vi "Get ixon camera info.vi"() -> ()   [LabVIEW 2011]
uses:
  <userlib>/atmcd32d.llb/HSSpeed_type typedef.ctl
  <userlib>/atmcd32d.llb/AndorCapabilities typedef.ctl
panel:
  out "Preamp gains":sgl[](array[numeric])
  out "# y pixels":i32
  out "# x pixels":i32
  out "highest EM gain":i32
  out "lowest EM gain":i32
  out "camera serial #":i32
  out "Flex version #":u32
  out "PCB version #":u32
  out "head model":string
  out "VS speeds":sgl[](array[numeric])
  out "fastest recommended VS speed":sgl format="%.2f"
  out "Camera capabilities":T1
  in  "EM?":T2
  out "HS Speeds on each channel":sgl[][](array[numeric])
  out "bit depth each channel":i32[](array[numeric])
  out "#preamp gains":i32
  out "# amplifiers":i32
  out "#ADC channels":i32
  out "Return from Initialize":u32
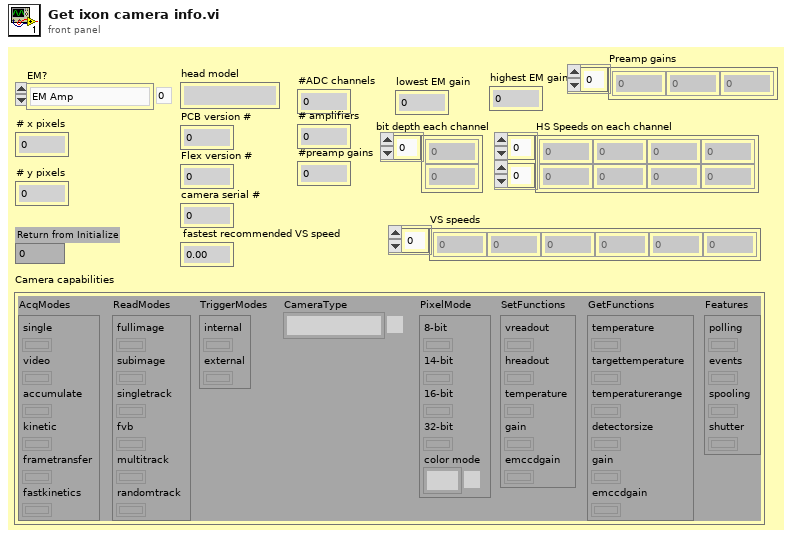
[diagram p1: front panel]
types:
  T1 = typedef "AndorCapabilities typedef.ctl" = cluster{"AcqModes":cluster{"single":bool, "video":bool, "accumulate":bool, "kinetic":bool, "frametransfer":bool, "fastkinetics":bool}, "ReadModes":cluster{"fullimage":bool, "subimage":bool, "singletrack":bool, "fvb":bool, "multitrack":bool, "randomtrack":bool}, "TriggerModes":cluster{"internal":bool, "external":bool}, "CameraType":enum32{"PDA", "iXon", "ICCD", "EMCCD", "CCD", "iStar", "third party camera"}, "PixelMode":cluster{"8-bit":bool, "14-bit":bool, "16-bit":bool, "32-bit":bool, "color mode":enum16{"Mono", "RGB", "CMY"}}, "SetFunctions":cluster{"vreadout":bool, "hreadout":bool, "temperature":bool, "gain":bool, "emccdgain":bool}, "GetFunctions":cluster{"temperature":bool, "targettemperature":bool, "temperaturerange":bool, "detectorsize":bool, "gain":bool, "emccdgain":bool}, "Features":cluster{"polling":bool, "events":bool, "spooling":bool, "shutter":bool}}
  T2 = typedef "HSSpeed_type typedef.ctl" = enum16{"EM Amp", "Conventional Amp"}
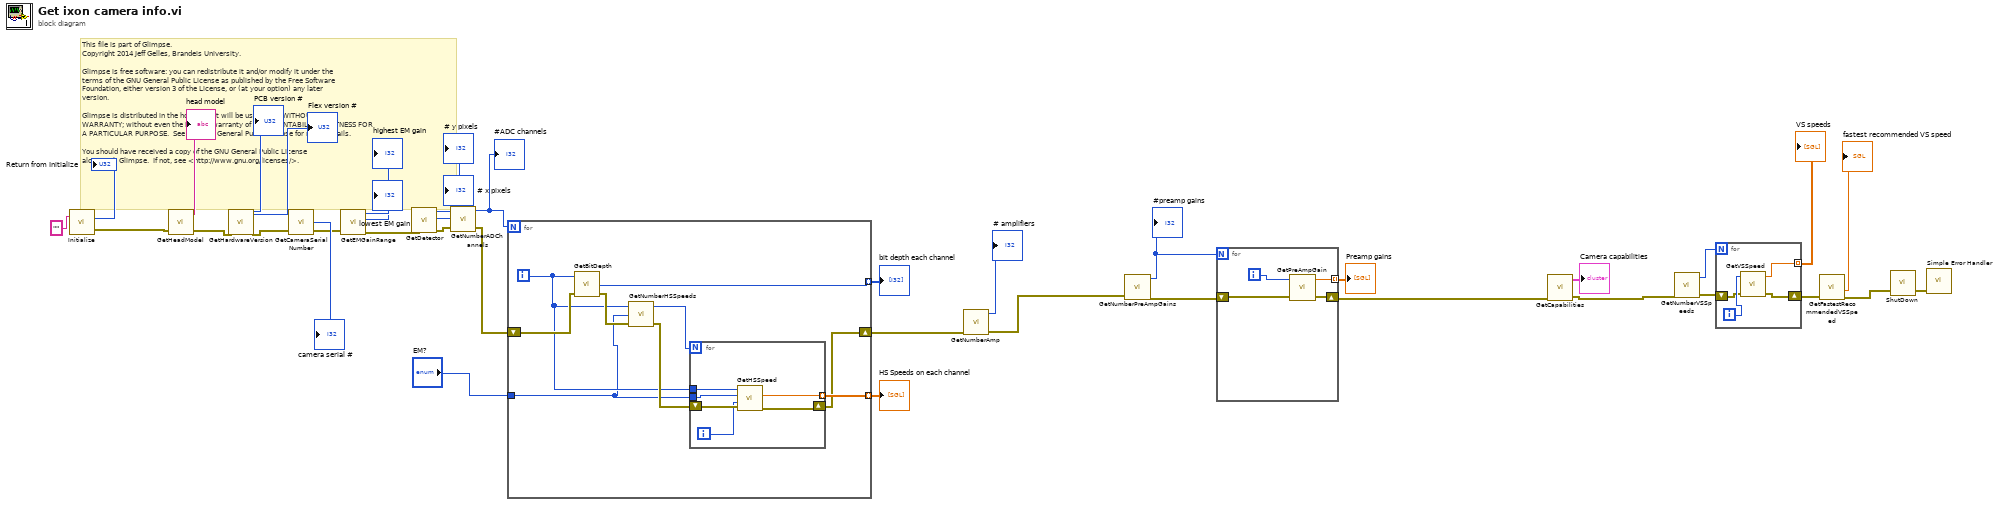
[diagram p0: block diagram]
diagram:
  # "This file is part of Glimpse. \nCopyright 2014 Jeff Gelles, Brandeis University.    \n\nGlimpse is free software: you can redistribute it and/or modify it under the \nterms of the GNU General Public License as published by the Free Software \nFoundation, either version 3 of the License, or (at your option) any later \nversion.\n\nGlimpse is distributed in the hope that it will be useful, but WITHOUT ANY \nWARRANTY; without even the implied warranty of MERCHANTABILITY or FITNESS FOR \nA PARTICULAR PURPOSE.  See the GNU General Public License for more details.\n\nYou should have received a copy of the GNU General Public License\nalong with Glimpse.  If not, see <http://www.gnu.org/licenses/>."
  n1 = call <userlib>:"Initialize.vi"("directory (\"\")"="" ("directory (\"\")")) -> ("error out"=w9:errorcluster, "DLL error code"=→"Return from Initialize":u32)  [unwired: 1 in]
  n2 = call <userlib>:"GetHeadModel.vi"("error in (no error)"=w9) -> ("error out"=w8:errorcluster, "model"=→"head model":string)  [unwired: 2 in, 1 out]
  n3 = call <userlib>:"GetHardwareVersion.vi"("error in (no error)"=w8) -> ("PCB"=→"PCB version #":u32, "Flex"=→"Flex version #":u32, "error out"=w7:errorcluster)  [unwired: 19 in, 5 out]
  n4 = call <userlib>:"GetCameraSerialNumber.vi"("error in (no error)"=w7) -> ("error out"=w6:errorcluster, "number"=→"camera serial #":i32)  [unwired: 2 in, 1 out]
  n5 = call <userlib>:"GetEMGainRange.vi"("error in (no error)"=w6) -> ("error out"=w5:errorcluster, "high"=→"highest EM gain":i32, "low"=→"lowest EM gain":i32)  [unwired: 3 in, 1 out]
  n6 = call <userlib>:"GetDetector.vi"("error in (no error)"=w5) -> ("error out"=w12:errorcluster, "ypixels"=→"# y pixels":i32, "xpixels"=→"# x pixels":i32)  [unwired: 3 in, 1 out]
  n7 = call <userlib>:"GetNumberADChannels.vi"("error in (no error)"=w12) -> ("error out"=w32:errorcluster, "number"=w33:i32)  [unwired: 2 in, 1 out]
  "#ADC channels" <- w33
  n8 = for {
    N: w33 -> [_]
    shift-right: [w40] -> w30
    shift-left: w32 -> [w46]
    tunnel: [w45] -> w31 mode=indexing
    tunnel: [w41] -> w28 mode=indexing
    tunnel: "EM?" -> [w38]
    i -> [w39]
    n9 = call <userlib>:"GetBitDepth.vi"("error in (no error)"=w46, "channel"=w39) -> ("error out"=w44:errorcluster, "depth"=w45:i32)  [unwired: 1 in, 1 out]
    n10 = call <userlib>:"GetNumberHSSpeeds.vi"("error in (no error)"=w44, "type"=w38, "channel"=w39) -> ("error out"=w43:errorcluster, "number"=w42:i32)  [unwired: 1 out]
    n11 = for {
      N: w42 -> [_]
      shift-right: [w50] -> w40
      shift-left: w43 -> [w52]
      tunnel: [w51] -> w41 mode=indexing
      tunnel: w39 -> [w49]
      tunnel: w38 -> [w48]
      i -> [w47]
      n12 = call <userlib>:"GetHSSpeed.vi"("error in (no error)"=w52, "index"=w47, "type"=w48, "channel"=w49) -> ("error out"=w50:errorcluster, "speed"=w51:sgl)  [unwired: 1 in, 1 out]
    }
  }
  "bit depth each channel" <- w31
  "HS Speeds on each channel" <- w28
  n13 = call <userlib>:"GetNumberAmp.vi"("error in (no error)"=w30) -> ("error out"=w29:errorcluster, "number"=→"# amplifiers":i32)  [unwired: 2 in, 1 out]
  n14 = call <userlib>:"GetNumberPreAmpGains.vi"("error in (no error)"=w29) -> ("error out"=w2:errorcluster, "number"=w4:i32)  [unwired: 2 in, 1 out]
  "#preamp gains" <- w4
  n15 = for {
    N: w4 -> [_]
    shift-right: [w55] -> w3
    shift-left: w2 -> [w54]
    tunnel: [w53] -> w1 mode=indexing
    i -> [w56]
    n16 = call <userlib>:"GetPreAmpGain.vi"("error in (no error)"=w54, "index"=w56) -> ("error out"=w55:errorcluster, "gain"=w53:sgl)  [unwired: 1 in, 1 out]
  }
  "Preamp gains" <- w1
  n17 = call <userlib>:"GetCapabilities.vi"("error in (no error)"=w3) -> ("error out"=w20:errorcluster, "caps"=→"Camera capabilities":T1)  [unwired: 2 in, 1 out]
  n18 = call <userlib>:"GetNumberVSSpeeds.vi"("error in (no error)"=w20) -> ("error out"=w21:errorcluster, "number"=w19:i32)  [unwired: 2 in, 1 out]
  n19 = for {
    N: w19 -> [_]
    tunnel: [w60] -> w23 mode=indexing
    shift-right: [w59] -> w22
    shift-left: w21 -> [w57]
    i -> [w58]
    n20 = call <userlib>:"GetVSSpeed.vi"("error in (no error)"=w57, "index"=w58) -> ("error out"=w59:errorcluster, "speed"=w60:sgl)  [unwired: 1 in, 1 out]
  }
  "VS speeds" <- w23
  n21 = call <userlib>:"GetFastestRecommendedVSSpeed.vi"("error in (no error)"=w22) -> ("error out"=w24:errorcluster, "speed"=→"fastest recommended VS speed":sgl)  [unwired: 3 in, 2 out]
  n22 = call <userlib>:"ShutDown.vi"("error in (no error)"=w24) -> ("error out"=w34:errorcluster)  [unwired: 1 in, 1 out]
  n23 = call <vilib>:"Simple Error Handler.vi"("error in (no error)"=w34) -> ()  [unwired: 4 in, 5 out]
